vi "Reset.vi"(8 "error in (no error)":errorcluster, 11 "vici_flow_actuator_parent in":refnum<class "heater_parent.lvclass">) -> (0 "error out":errorcluster, 3 "vici_flow_actuator_parent out":refnum<class "heater_parent.lvclass">)   [LabVIEW 2020, in "polar_bear_plus_drivers.lvlib" / "heater_parent.lvclass"]
doc: "Resets the instrument and provides some default setup commands. For the moment this is the same as the Default Instrument Setup VI."
uses:
  <instrlib>/RxnRover/Driver Polar Bear Plus/heater_parent/heater_parent.lvclass
  <instrlib>/RxnRover/Driver Polar Bear Plus/heater_parent/heater_parent.lvclass/heater_parent.ctl
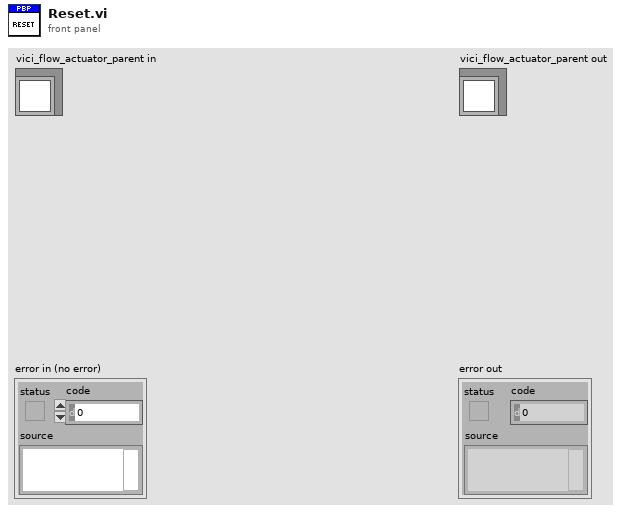
[diagram p1: front panel]
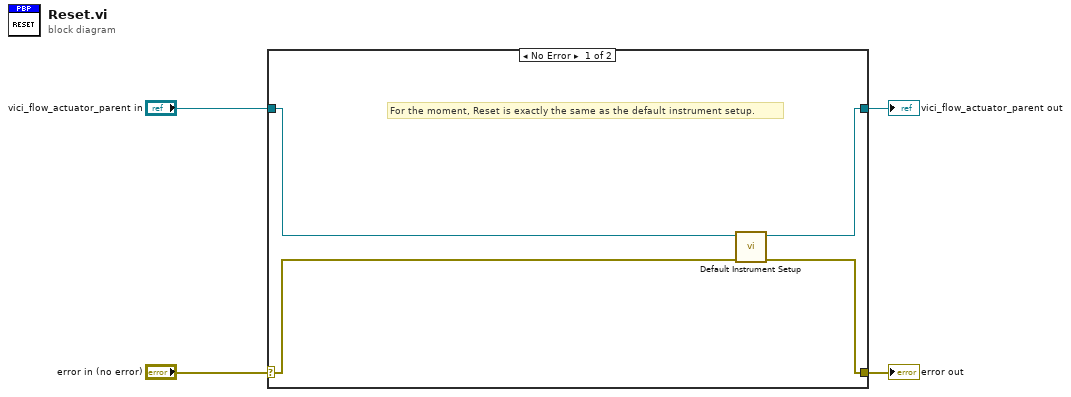
[diagram p0: block diagram]
diagram:
  n1 = case shown="No Error" "error in (no error)" {
    selector: "error in (no error)" -> [w7 w10]
    tunnel: [w6 w10] -> w3
    tunnel: [w5 w9] -> w1
    tunnel: "vici_flow_actuator_parent in" -> [w8 w9]
    frame No Error {
      # "For the moment, Reset is exactly the same as the default instrument setup."
      n2 = call-dynamic "Default Instrument Setup.vi"("error in (no error)"=w7, "heater_parent in"=w8) -> ("error out"=w6:errorcluster, "heater_parent out"=w5:refnum<class "heater_parent.lvclass">)  [unwired: 8 in]
    }
    frame Error {
    }
  }
  "error out" <- w3
  "vici_flow_actuator_parent out" <- w1
